vi "Combination_Digitizer_Configure.vi"(0 "Mode":T1(ring), 1 "Horizontal Settings":T2={"number of records"=1, "reference position"=50.0, "min record length"=50000, "min sample rate"=200000.0, "enforce realtime"=FALSE, "maximum input frequency"=0.0} {"maximum input frequency" format="%.2f"; "min sample rate" step=1000000.0 format="%.0p"; "reference position" format="%.1f"; "number of records" step=1}, 2 "Vertical Settings":T4={"vertical coupling"=enum."DC", "probe attenuation"=20.0, "vertical range"=120.0, "vertical offset"=0.0} {"vertical offset" format="%.4f"; "vertical range" format="%.2f"; "probe attenuation" format="%.1f"}, 3 "Trigger settings":T3={"trigger level"=30.0, "trigger type"=enum."Edge", "Trigger Source"=enum."Channel 0", "Trigger Slope"=enum."Positive"} {"trigger level" format="%.2f"}, 5 "Channel Name":string="0", 11 "error in":errorcluster) -> (6 "Waveform Array":waveform(dbl)[](array[waveform]), 8 "Ch1_Plot":dbl[](array[numeric]), 15 "error out":errorcluster)   [LabVIEW 2010]
uses:
  <instrlib>/niScope/Controls/niScope trigger slope.ctl
  <instrlib>/niScope/Controls/niScope trigger source.ctl
  <instrlib>/niScope/Controls/niScope export destinations.ctl
  <instrlib>/niScope/Controls/niScope exportable signals.ctl
  <instrlib>/niScope/Controls/niScope trigger source digital.ctl
  <instrlib>/niScope/Configure/Trigger/niScope Configure Trigger Edge.vi
  <instrlib>/niScope/Configure/Trigger/niScope Configure Trigger Digital.vi
  <instrlib>/niScope/Configure/Trigger/niScope Configure Trigger Immediate.vi
  <instrlib>/niScope/Acquire/niScope Multi Read Cluster.vi
  <instrlib>/niScope/Acquire/Fetch/niScope Multi Fetch Cluster.vi
panel:
  out "Waveform":T5(graph)
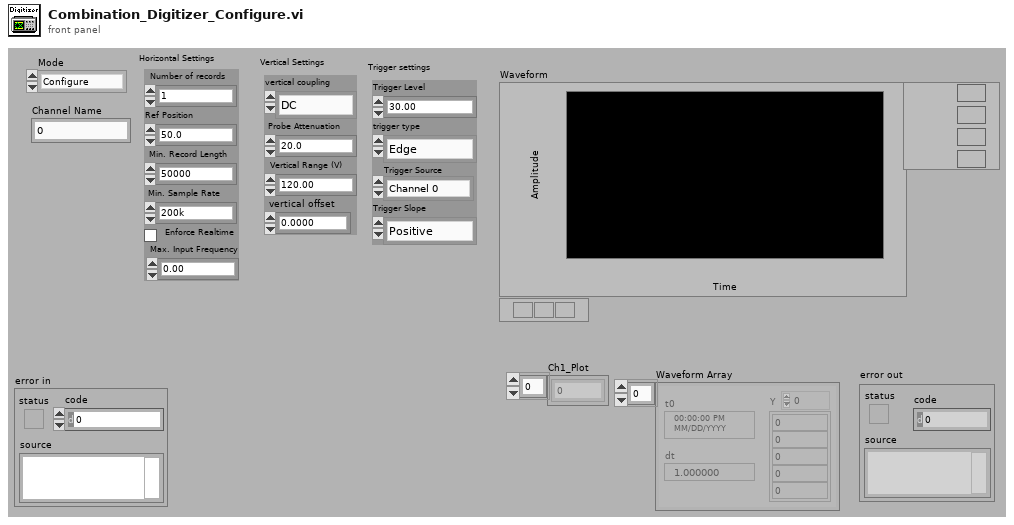
[diagram p1: front panel]
types:
  T1 = enum16{"Configure", "Read", "TriggerRead", "Close", "Init"}
  T2 = cluster{"number of records":i32, "reference position":dbl, "min record length":i32, "min sample rate":dbl, "enforce realtime":bool, "maximum input frequency":dbl}
  T3 = cluster{"trigger level":dbl, "trigger type":enum16{"Edge", "Digital", "Immediate"}, "Trigger Source":enum8{"Immediate", "Channel 0", "Channel 1", "Channel 2", "Channel 3", "Channel 4", "Channel 5", "Channel 6", "Channel 7", "External TRIG", "Software Trigger", "RTSI 0", "RTSI 1", "RTSI 2", "RTSI 3", "RTSI 4", "RTSI 5", "RTSI 6", "PFI 0", "PFI 1", "PFI 2", "PXI Star Trigger"}, "Trigger Slope":enum16{"Positive", "Negative"}}
  T4 = cluster{"vertical coupling":enum16{"AC", "DC", "Ground"}, "probe attenuation":dbl, "vertical range":dbl, "vertical offset":dbl}
  T5 = cluster{"relativeInitialX":dbl, "xIncrement":dbl, "wfm":dbl[]}[]
  T6 = typedef "niScope trigger source.ctl" = string
  T7 = typedef "niScope trigger source digital.ctl" = string
  T8 = typedef "niScope export destinations.ctl" = string
  T9 = cluster{"Dig1 Channels":string, "Channel1 Scale":dbl, "Dig1 Used":bool, "Dig1 Ref":refnum<k15>, "min record length":i32, "Dig2 Channels":string, "Dig2 Used":bool, "Dig2 Ref":refnum<k15>, "trigger type":enum16{"Edge", "Digital", "Immediate"}}
  T10 = enum8{"Immediate", "Channel 0", "Channel 1", "Channel 2", "Channel 3", "Channel 4", "Channel 5", "Channel 6", "Channel 7", "External TRIG", "Software Trigger", "RTSI 0", "RTSI 1", "RTSI 2", "RTSI 3", "RTSI 4", "RTSI 5", "RTSI 6", "PFI 0", "PFI 1", "PFI 2", "PXI Star Trigger"}
  T11 = typedef "niScope trigger slope.ctl" = i32
  T12 = typedef "niScope exportable signals.ctl" = u16
  T13 = cluster{"relativeInitialX":dbl, "xIncrement":dbl, "wfm":dbl[]}
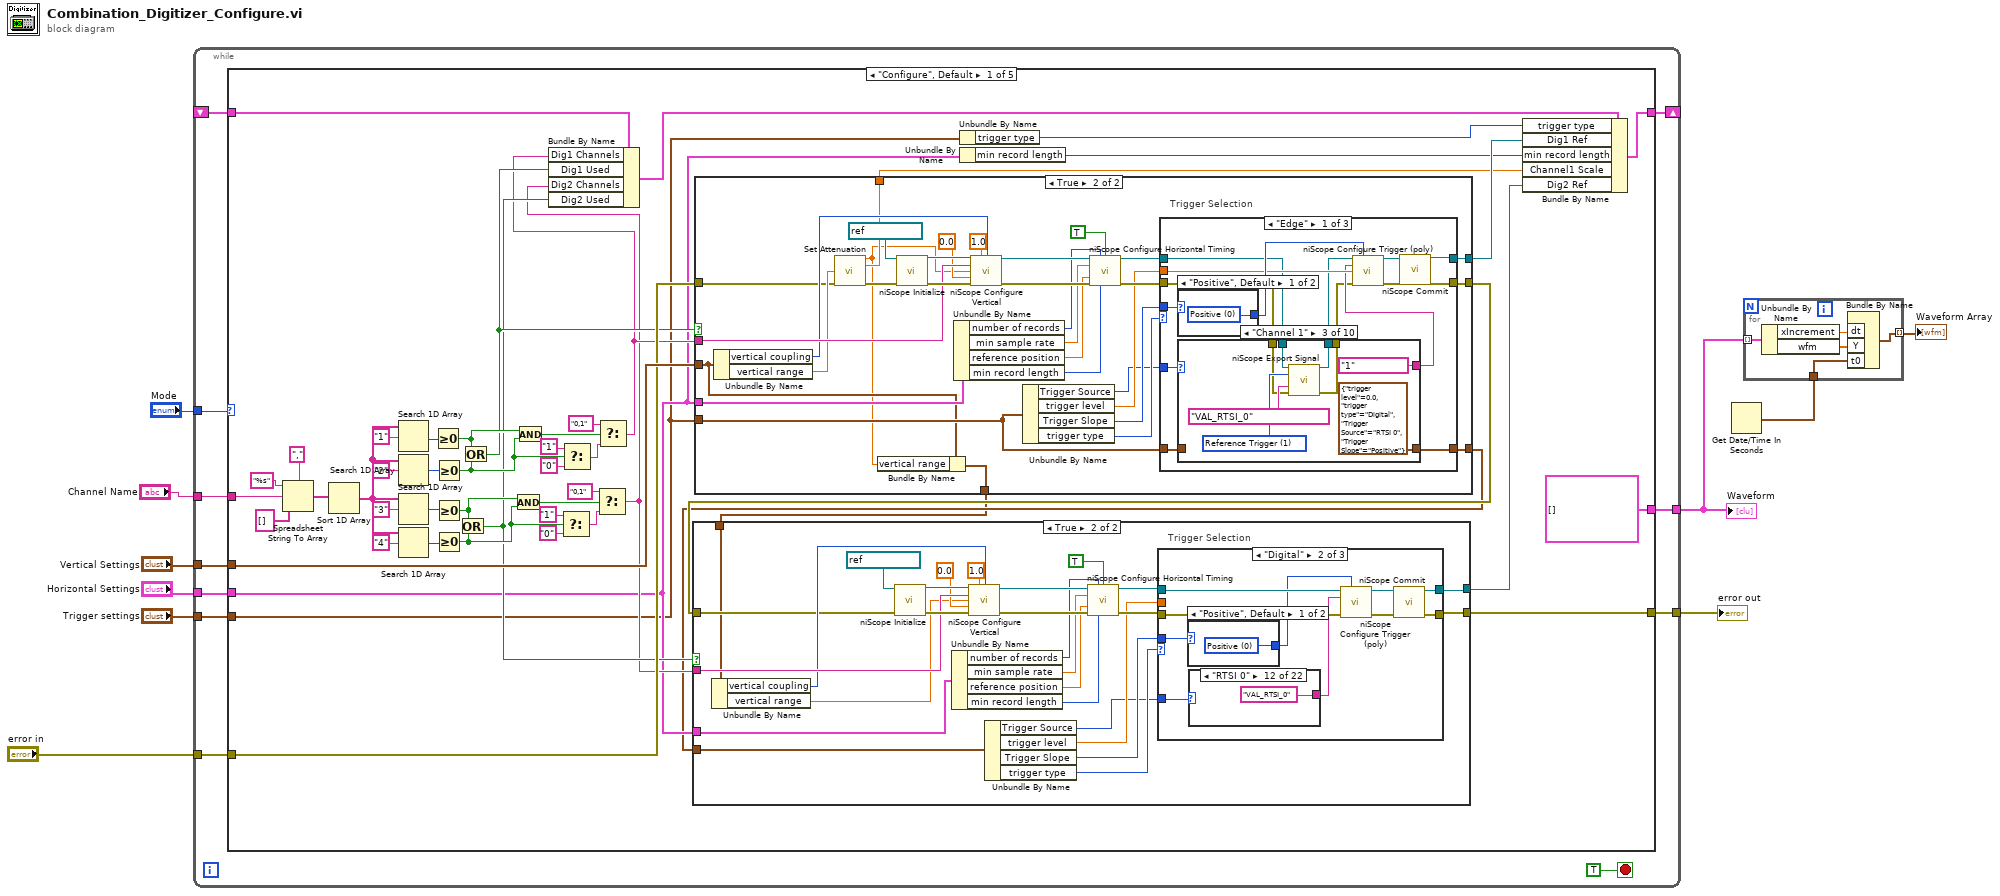
[diagram p0: block diagram]
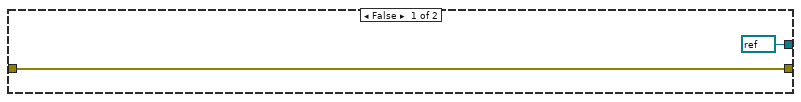
[diagram p2: hidden frame]
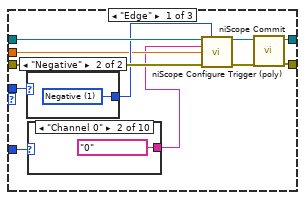
[diagram p3: hidden frame]
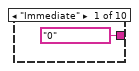
[diagram p4: hidden frame]
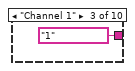
[diagram p5: hidden frame]
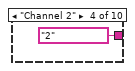
[diagram p6: hidden frame]
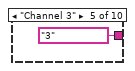
[diagram p7: hidden frame]
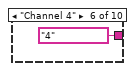
[diagram p8: hidden frame]
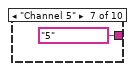
[diagram p9: hidden frame]
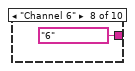
[diagram p10: hidden frame]
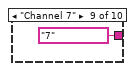
[diagram p11: hidden frame]
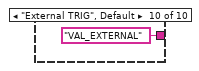
[diagram p12: hidden frame]
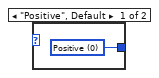
[diagram p13: hidden frame]
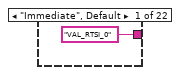
[diagram p14: hidden frame]
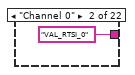
[diagram p15: hidden frame]
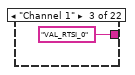
[diagram p16: hidden frame]
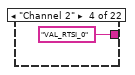
[diagram p17: hidden frame]
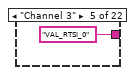
[diagram p18: hidden frame]
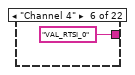
[diagram p19: hidden frame]
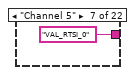
[diagram p20: hidden frame]
diagram:
  n1 = while {
    tunnel: "Mode" -> [w20]
    shift-right: [w14] -> _
    shift-left: _ -> [w19]
    tunnel: "error in" -> [w13]
    tunnel: "Channel Name" -> [w18]
    tunnel: "Vertical Settings" -> [w17]
    tunnel: "Horizontal Settings" -> [w16]
    tunnel: "Trigger settings" -> [w15]
    tunnel: [w12] -> w5
    tunnel: [w11] -> w3
    stop <- TRUE stop-if-true
    n2 = case shown="\"Configure\", Default" w20 {
      tunnel: w19 -> [w38 w307 w410 w437 w486]
      tunnel: w18 -> [w42 _ _ _ _]
      tunnel: w17 -> [w41 _ _ _ _]
      tunnel: w16 -> [w28 _ _ _ _]
      tunnel: w15 -> [w25 _ _ _ _]
      tunnel: [w40 w307 w410 w437 T9 {"Dig1 Channels"="", "Channel1 Scale"=0.0, "Dig1 Used"=FALSE, "Dig1 Ref"="", "min record length"=0, "Dig2 Channels"="", "Dig2 Used"=FALSE, "Dig2 Ref"="", "trigger type"=enum."Immediate"}] -> w14
      tunnel: w13 -> [w39 w313 w413 w443 w489]
      tunnel: [w33 w318 w416 w448 w492] -> w12
      tunnel: [T5 [] w305 T5 [] w436 T5 []] -> w11
      frame "Configure", Default {
        n3 = Spreadsheet String To Array(delimiter (Tab)=",", format string="%s", spreadsheet string=w42, array type (2D Dbl)=string[] []) -> (array=w67:string[])
        n4 = Sort 1D Array(array=w67) -> (sorted array=w66:string[])
        n5 = Search 1D Array(1D array=w66, element="1") -> (index of element=w61:i32)  [unwired: 1 in]
        n6 = Search 1D Array(1D array=w66, element="2") -> (index of element=w58:i32)  [unwired: 1 in]
        n7 = Search 1D Array(1D array=w66, element="3") -> (index of element=w59:i32)  [unwired: 1 in]
        n8 = Search 1D Array(1D array=w66, element="4") -> (index of element=w60:i32)  [unwired: 1 in]
        n9 = Greater Or Equal To 0?(x=w61) -> (x >= 0?=w57:bool)
        n10 = Greater Or Equal To 0?(x=w58) -> (x >= 0?=w53:bool)
        n11 = Greater Or Equal To 0?(x=w59) -> (x >= 0?=w56:bool)
        n12 = Greater Or Equal To 0?(x=w60) -> (x >= 0?=w44:bool)
        n13 = Or(x=w56, y=w44) -> (x .or. y?=w31:bool)
        n14 = Or(x=w57, y=w53) -> (x .or. y?=w32:bool)
        n15 = And(x=w56, y=w44) -> (x .and. y?=w45:bool)
        n16 = And(x=w57, y=w53) -> (x .and. y?=w55:bool)
        n17 = Select(t="1", s=w44, f="0") -> (s? t:f=w47:string)
        n18 = Select(t="1", s=w53, f="0") -> (s? t:f=w51:string)
        n19 = Select(t="0,1", s=w45, f=w47) -> (s? t:f=w29:string)
        n20 = Select(t="0,1", s=w55, f=w51) -> (s? t:f=w30:string)
        n21 = Bundle By Name(cluster=w38, "Dig1 Channels"=w30, "Dig1 Used"=w32, "Dig2 Channels"=w29, "Dig2 Used"=w31) -> (w37:T9)
        n22 = case shown="True" w32 {
          tunnel: [w165 w193] -> w43
          tunnel: w39 -> [w165 w187]
          tunnel: w30 -> [_ w191]
          tunnel: w41 -> [w161 w168]
          tunnel: w28 -> [_ w182]
          tunnel: w25 -> [w162 w170]
          tunnel: [refnum<k15> refnum ("instrument handle out") w176] -> w36
          tunnel: [1.0 ("Gain Multiplier") w174] -> w34
          tunnel: [w162 w169] -> w23
          tunnel: [w161 w166] -> w22
          frame False {
          }
          frame True {
            n23 = Unbundle By Name(w168) -> ("vertical coupling"=w190:enum16{"AC", "DC", "Ground"}, "vertical range"=w188:dbl)
            n24 = call "Set Attenuation.vi"("vertical range"=w188, "error in"=w187) -> ("Requested Range"=w167:dbl, "Gain Multiplier"=w174:dbl, "error out"=w186:errorcluster)  [unwired: 11 in]
            n25 = Bundle By Name(cluster=w168, "vertical range"=w167) -> (w166:T4)
            n26 = call <instrlib>:"niScope Initialize.vi"("resource name"=refnum<k15> "PXI1Slot6", "error in"=w186) -> ("instrument handle"=w197:refnum<k15>, "error out"=w194:errorcluster)  [unwired: 12 in]
            n27 = Unbundle By Name(w182) -> ("number of records"=w181:i32, "min sample rate"=w180:dbl, "reference position"=w179:dbl, "min record length"=w178:i32)
            n28 = call <instrlib>:"niScope Configure Vertical.vi"("instrument handle"=w197, "probe attenuation"=1.0, "vertical coupling"=w190, "channels"=w191, "vertical range"=w167, "vertical offset"=0.0, "error in"=w194) -> ("instrument handle out"=w184:refnum<k15>, "error out"=w183:errorcluster)  [unwired: 7 in]
            n29 = Unbundle By Name(w170) -> ("Trigger Source"=w171:T10, "trigger level"=w177:dbl, "Trigger Slope"=w172:enum16{"Positive", "Negative"}, "trigger type"=w173:enum16{"Edge", "Digital", "Immediate"})
            n30 = call <instrlib>:"niScope Configure Horizontal Timing.vi"("instrument handle"=w184, "number of records"=w181, "enforce realtime"=TRUE, "min sample rate"=w180, "reference position"=w179, "error in"=w183, "min record length"=w178) -> ("instrument handle out"=w195:refnum<k15>, "error out"=w196:errorcluster)  [unwired: 7 in]
            n31 = case "Trigger Selection" shown="\"Edge\"" w173 {
              tunnel: w196 -> [w199 w271 w300]
              tunnel: [w204 w264 w297] -> w193
              tunnel: w195 -> [w201 w270 w299]
              tunnel: [w205 w265 w298] -> w176
              tunnel: w171 -> [w209 w267 _]
              tunnel: w177 -> [w210 _ _]
              tunnel: w172 -> [w212 w269 _]
              tunnel: w170 -> [w203 w263 w296]
              tunnel: [w202 w263 w296] -> w169
              frame "Edge" {
                n32 = case shown="\"Positive\", Default" w212 {
                  tunnel: [w261 w262] -> w211
                  frame "Positive", Default {
                    w261 = T11 0 items=["Positive", "Negative"] ("trigger slope")
                  }
                  frame "Negative" {
                    w262 = T11 1 items=["Positive", "Negative"] ("trigger slope")
                  }
                }
                n33 = case shown="\"Channel 1\"" w209 {
                  tunnel: [T6 "0" ("trigger source") T6 "0" ("trigger source") T6 "1" ("trigger source") T6 "2" ("trigger source") T6 "3" ("trigger source") T6 "4" ("trigger source") T6 "5" ("trigger source") T6 "6" ("trigger source") T6 "7" ("trigger source") T6 "VAL_EXTERNAL" ("trigger source")] -> w208
                  tunnel: w203 -> [w215 _ _ w235 w239 w243 w247 w251 w255 w259]
                  tunnel: [w215 T3 {"trigger level"=0.0, "trigger type"=enum."Digital", "Trigger Source"=enum."RTSI 0", "Trigger Slope"=enum."Positive"} ("Trigger settings") T3 {"trigger level"=0.0, "trigger type"=enum."Digital", "Trigger Source"=enum."RTSI 0", "Trigger Slope"=enum."Positive"} ("Trigger settings") w235 w239 w243 w247 w251 w255 w259] -> w202
                  tunnel: w201 -> [w214 w220 w228 w234 w238 w242 w246 w250 w254 w258]
                  tunnel: [w214 w218 w227 w234 w238 w242 w246 w250 w254 w258] -> w200
                  tunnel: w199 -> [w213 w219 w226 w233 w237 w241 w245 w249 w253 w257]
                  tunnel: [w213 w217 w225 w233 w237 w241 w245 w249 w253 w257] -> w198
                  frame "Immediate" {
                  }
                  frame "Channel 0" {
                    w221 = T12 1 items=["None"=0, "Start Trigger"=2, "Advance Trigger"=5, "Reference Trigger"=1, "End of Record Event"=4, "End of Acquisition Event"=3, "Ready for Start Event"=7, "Ready for Advance Event"=6, "Ready for Reference Event"=10, "Reference Clock"=100, "Sample Clock"=101, "5 Volt Power"=13] ("signal")
                    n34 = call <instrlib>:"niScope Export Signal.vi"("instrument handle"=w220, "signal"=w221, "output terminal"=T8 "VAL_RTSI_0", "error in"=w219) -> ("instrument handle out"=w218:refnum<k15>, "error out"=w217:errorcluster)  [unwired: 10 in]
                  }
                  frame "Channel 1" {
                    w229 = T12 1 items=["None"=0, "Start Trigger"=2, "Advance Trigger"=5, "Reference Trigger"=1, "End of Record Event"=4, "End of Acquisition Event"=3, "Ready for Start Event"=7, "Ready for Advance Event"=6, "Ready for Reference Event"=10, "Reference Clock"=100, "Sample Clock"=101, "5 Volt Power"=13] ("signal")
                    n35 = call <instrlib>:"niScope Export Signal.vi"("instrument handle"=w228, "signal"=w229, "output terminal"=T8 "VAL_RTSI_0", "error in"=w226) -> ("instrument handle out"=w227:refnum<k15>, "error out"=w225:errorcluster)  [unwired: 10 in]
                  }
                  frame "Channel 2" {
                  }
                  frame "Channel 3" {
                  }
                  frame "Channel 4" {
                  }
                  frame "Channel 5" {
                  }
                  frame "Channel 6" {
                  }
                  frame "Channel 7" {
                  }
                  frame "External TRIG", Default {
                  }
                }
                n36 = call-poly <instrlib>:"niScope Configure Trigger (poly).vi"("instrument handle"=w200, "trigger slope"=w211, "trigger source"=w208, "trigger level"=w210, "error in"=w198) -> ("instrument handle out"=w207:refnum<k15>, "error out"=w206:errorcluster)  [unwired: 9 in]
                n37 = call <instrlib>:"niScope Commit.vi"("instrument handle"=w207, "error in"=w206) -> ("instrument handle out"=w205:refnum<k15>, "error out"=w204:errorcluster)  [unwired: 12 in]
              }
              frame "Digital" {
                n38 = case shown="\"Negative\"" w269 {
                  tunnel: [w294 w295] -> w268
                  frame "Positive", Default {
                    w294 = T11 0 items=["Positive", "Negative"] ("trigger slope")
                  }
                  frame "Negative" {
                    w295 = T11 1 items=["Positive", "Negative"] ("trigger slope")
                  }
                }
                n39 = case shown="\"PXI Star Trigger\"" w267 {
                  tunnel: [T7 "VAL_RTSI_0" ("trigger source") T7 "VAL_RTSI_0" ("trigger source") T7 "VAL_RTSI_0" ("trigger source") T7 "VAL_RTSI_0" ("trigger source") T7 "VAL_RTSI_0" ("trigger source") T7 "VAL_RTSI_0" ("trigger source") T7 "VAL_RTSI_0" ("trigger source") T7 "VAL_RTSI_0" ("trigger source") T7 "VAL_RTSI_0" ("trigger source") T7 "VAL_RTSI_0" ("trigger source") T7 "VAL_RTSI_0" ("trigger source") T7 "VAL_RTSI_0" ("trigger source") T7 "VAL_RTSI_1" ("trigger source") T7 "VAL_RTSI_2" ("trigger source") T7 "VAL_RTSI_3" ("trigger source") T7 "VAL_RTSI_4" ("trigger source") T7 "VAL_RTSI_5" ("trigger source") T7 "VAL_RTSI_6" ("trigger source") T7 "VAL_PFI_0" ("trigger source") T7 "VAL_PFI_1" ("trigger source") T7 "VAL_PFI_2" ("trigger source") T7 "VAL_PXI_STAR" ("trigger source")] -> w266
                  frame "Immediate", Default {
                  }
                  frame "Channel 0" {
                  }
                  frame "Channel 1" {
                  }
                  frame "Channel 2" {
                  }
                  frame "Channel 3" {
                  }
                  frame "Channel 4" {
                  }
                  frame "Channel 5" {
                  }
                  frame "Channel 6" {
                  }
                  frame "Channel 7" {
                  }
                  frame "External TRIG" {
                  }
                  frame "Software Trigger" {
                  }
                  frame "RTSI 0" {
                  }
                  frame "RTSI 1" {
                  }
                  frame "RTSI 2" {
                  }
                  frame "RTSI 3" {
                  }
                  frame "RTSI 4" {
                  }
                  frame "RTSI 5" {
                  }
                  frame "RTSI 6" {
                  }
                  frame "PFI 0" {
                  }
                  frame "PFI 1" {
                  }
                  frame "PFI 2" {
                  }
                  frame "PXI Star Trigger" {
                  }
                }
                n40 = call-poly <instrlib>:"niScope Configure Trigger (poly).vi"("instrument handle"=w270, "trigger slope"=w268, "trigger source"=w266, "error in"=w271) -> ("instrument handle out"=w265:refnum<k15>, "error out"=w264:errorcluster)  [unwired: 10 in]
              }
              frame "Immediate", Default {
                n41 = call-poly <instrlib>:"niScope Configure Trigger (poly).vi"("instrument handle"=w299, "error in"=w300) -> ("instrument handle out"=w298:refnum<k15>, "error out"=w297:errorcluster)  [unwired: 12 in]
              }
            }
          }
        }
        n42 = case shown="True" w31 {
          tunnel: [w72 w79] -> w33
          tunnel: w43 -> [w72 w84]
          tunnel: w29 -> [_ w96]
          tunnel: w28 -> [_ w90]
          tunnel: w23 -> [_ w85]
          tunnel: [refnum<k15> refnum ("instrument handle out") w80] -> w35
          tunnel: w22 -> [_ w73]
          frame False {
          }
          frame True {
            n43 = Unbundle By Name(w73) -> ("vertical coupling"=w95:enum16{"AC", "DC", "Ground"}, "vertical range"=w83:dbl)
            n44 = call <instrlib>:"niScope Initialize.vi"("resource name"=refnum<k15> "PXI1Slot4", "error in"=w84) -> ("instrument handle"=w99:refnum<k15>, "error out"=w98:errorcluster)  [unwired: 12 in]
            n45 = Unbundle By Name(w90) -> ("number of records"=w89:i32, "min sample rate"=w88:dbl, "reference position"=w87:dbl, "min record length"=w86:i32)
            n46 = call <instrlib>:"niScope Configure Vertical.vi"("instrument handle"=w99, "probe attenuation"=1.0, "vertical coupling"=w95, "channels"=w96, "vertical range"=w83, "vertical offset"=0.0, "error in"=w98) -> ("instrument handle out"=w92:refnum<k15>, "error out"=w91:errorcluster)  [unwired: 7 in]
            n47 = Unbundle By Name(w85) -> ("Trigger Source"=w74:T10, "trigger level"=w77:dbl, "Trigger Slope"=w75:enum16{"Positive", "Negative"}, "trigger type"=w76:enum16{"Edge", "Digital", "Immediate"})
            n48 = call <instrlib>:"niScope Configure Horizontal Timing.vi"("instrument handle"=w92, "number of records"=w89, "enforce realtime"=TRUE, "min sample rate"=w88, "reference position"=w87, "error in"=w91, "min record length"=w86) -> ("instrument handle out"=w81:refnum<k15>, "error out"=w78:errorcluster)  [unwired: 7 in]
            n49 = case "Trigger Selection" shown="\"Digital\"" w76 {
              tunnel: w78 -> [w110 w132 w160]
              tunnel: [w100 w123 w157] -> w79
              tunnel: w81 -> [w109 w131 w159]
              tunnel: [w102 w124 w158] -> w80
              tunnel: w74 -> [w105 w128 _]
              tunnel: w77 -> [w106 _ _]
              tunnel: w75 -> [w108 w130 _]
              frame "Edge" {
                n50 = case shown="\"Negative\"" w108 {
                  tunnel: [w121 w122] -> w107
                  frame "Positive", Default {
                    w121 = T11 0 items=["Positive", "Negative"] ("trigger slope")
                  }
                  frame "Negative" {
                    w122 = T11 1 items=["Positive", "Negative"] ("trigger slope")
                  }
                }
                n51 = case shown="\"Channel 0\"" w105 {
                  tunnel: [T6 "0" ("trigger source") T6 "0" ("trigger source") T6 "1" ("trigger source") T6 "2" ("trigger source") T6 "3" ("trigger source") T6 "4" ("trigger source") T6 "5" ("trigger source") T6 "6" ("trigger source") T6 "7" ("trigger source") T6 "VAL_EXTERNAL" ("trigger source")] -> w104
                  frame "Immediate" {
                  }
                  frame "Channel 0" {
                  }
                  frame "Channel 1" {
                  }
                  frame "Channel 2" {
                  }
                  frame "Channel 3" {
                  }
                  frame "Channel 4" {
                  }
                  frame "Channel 5" {
                  }
                  frame "Channel 6" {
                  }
                  frame "Channel 7" {
                  }
                  frame "External TRIG", Default {
                  }
                }
                n52 = call-poly <instrlib>:"niScope Configure Trigger (poly).vi"("instrument handle"=w109, "trigger slope"=w107, "trigger source"=w104, "trigger level"=w106, "error in"=w110) -> ("instrument handle out"=w103:refnum<k15>, "error out"=w101:errorcluster)  [unwired: 9 in]
                n53 = call <instrlib>:"niScope Commit.vi"("instrument handle"=w103, "error in"=w101) -> ("instrument handle out"=w102:refnum<k15>, "error out"=w100:errorcluster)  [unwired: 12 in]
              }
              frame "Digital" {
                n54 = case shown="\"Positive\", Default" w130 {
                  tunnel: [w155 w156] -> w129
                  frame "Positive", Default {
                    w155 = T11 0 items=["Positive", "Negative"] ("trigger slope")
                  }
                  frame "Negative" {
                    w156 = T11 1 items=["Positive", "Negative"] ("trigger slope")
                  }
                }
                n55 = case shown="\"RTSI 0\"" w128 {
                  tunnel: [T7 "VAL_RTSI_0" ("trigger source") T7 "VAL_RTSI_0" ("trigger source") T7 "VAL_RTSI_0" ("trigger source") T7 "VAL_RTSI_0" ("trigger source") T7 "VAL_RTSI_0" ("trigger source") T7 "VAL_RTSI_0" ("trigger source") T7 "VAL_RTSI_0" ("trigger source") T7 "VAL_RTSI_0" ("trigger source") T7 "VAL_RTSI_0" ("trigger source") T7 "VAL_RTSI_0" ("trigger source") T7 "VAL_RTSI_0" ("trigger source") T7 "VAL_RTSI_0" ("trigger source") T7 "VAL_RTSI_1" ("trigger source") T7 "VAL_RTSI_2" ("trigger source") T7 "VAL_RTSI_3" ("trigger source") T7 "VAL_RTSI_4" ("trigger source") T7 "VAL_RTSI_5" ("trigger source") T7 "VAL_RTSI_6" ("trigger source") T7 "VAL_PFI_0" ("trigger source") T7 "VAL_PFI_1" ("trigger source") T7 "VAL_PFI_2" ("trigger source") T7 "VAL_PXI_STAR" ("trigger source")] -> w127
                  frame "Immediate", Default {
                  }
                  frame "Channel 0" {
                  }
                  frame "Channel 1" {
                  }
                  frame "Channel 2" {
                  }
                  frame "Channel 3" {
                  }
                  frame "Channel 4" {
                  }
                  frame "Channel 5" {
                  }
                  frame "Channel 6" {
                  }
                  frame "Channel 7" {
                  }
                  frame "External TRIG" {
                  }
                  frame "Software Trigger" {
                  }
                  frame "RTSI 0" {
                  }
                  frame "RTSI 1" {
                  }
                  frame "RTSI 2" {
                  }
                  frame "RTSI 3" {
                  }
                  frame "RTSI 4" {
                  }
                  frame "RTSI 5" {
                  }
                  frame "RTSI 6" {
                  }
                  frame "PFI 0" {
                  }
                  frame "PFI 1" {
                  }
                  frame "PFI 2" {
                  }
                  frame "PXI Star Trigger" {
                  }
                }
                n56 = call-poly <instrlib>:"niScope Configure Trigger (poly).vi"("instrument handle"=w131, "trigger slope"=w129, "trigger source"=w127, "error in"=w132) -> ("instrument handle out"=w126:refnum<k15>, "error out"=w125:errorcluster)  [unwired: 10 in]
                n57 = call <instrlib>:"niScope Commit.vi"("instrument handle"=w126, "error in"=w125) -> ("instrument handle out"=w124:refnum<k15>, "error out"=w123:errorcluster)  [unwired: 12 in]
              }
              frame "Immediate", Default {
                n58 = call-poly <instrlib>:"niScope Configure Trigger (poly).vi"("instrument handle"=w159, "error in"=w160) -> ("instrument handle out"=w158:refnum<k15>, "error out"=w157:errorcluster)  [unwired: 12 in]
              }
            }
          }
        }
        n59 = Unbundle By Name(w25) -> ("trigger type"=w24:enum16{"Edge", "Digital", "Immediate"})
        n60 = Unbundle By Name(w28) -> ("min record length"=w27:i32)
        n61 = Bundle By Name(cluster=w37, "trigger type"=w24, "Dig1 Ref"=w36, "min record length"=w27, "Channel1 Scale"=w34, "Dig2 Ref"=w35) -> (w40:T9)
      }
      frame "Read" {
        n62 = Unbundle By Name(w307) -> ("trigger type"=w302:enum16{"Edge", "Digital", "Immediate"}, "Dig1 Used"=w317:bool, "Dig1 Ref"=w316:refnum<k15>, "Dig1 Channels"=w315:string, "min record length"=w314:i32, "Channel1 Scale"=w308:dbl)
        n63 = Unbundle By Name(w307) -> ("trigger type"=w301:enum16{"Edge", "Digital", "Immediate"}, "Dig2 Used"=w312:bool, "Dig2 Ref"=w311:refnum<k15>, "Dig2 Channels"=w310:string, "min record length"=w309:i32)
        n64 = case shown="True" w317 {
          tunnel: w315 -> [_ w381]
          tunnel: w313 -> [w375 w379]
          tunnel: w316 -> [_ w382]
          tunnel: [w375 w377] -> w319
          tunnel: [T5 [] ("waveform") w378] -> w320
          tunnel: w314 -> [_ w380]
          tunnel: w302 -> [_ w376]
          frame False {
          }
          frame True {
            n65 = case shown="\"Digital\", Default" w376 {
              tunnel: w382 -> [w389 w399]
              tunnel: w381 -> [w388 w398]
              tunnel: w380 -> [w387 w397]
              tunnel: w379 -> [w386 w396]
              tunnel: [w384 w391] -> w378
              tunnel: [w383 w394] -> w377
              frame "Immediate" {
                n66 = call-poly <instrlib>:"niScope Read (poly).vi"("timeout"=10.0, "error in"=w386, "numSamples"=w387, "channels"=w388, "instrument handle"=w389) -> ("error out"=w383:errorcluster, "waveform"=w384:T5)  [unwired: 3 in, 2 out]
              }
              frame "Digital", Default {
                n67 = call-poly <instrlib>:"niScope Fetch (poly).vi"("timeout"=10.0, "error in"=w396, "numSamples"=w397, "channels"=w398, "instrument handle"=w399) -> ("error out"=w393:errorcluster, "waveform"=w392:T5, "instrument handle out"=w390:refnum<k15>)  [unwired: 3 in, 1 out]
                n68 = case shown="Error" w393 {
                  tunnel: w393 -> [w400 w406]
                  tunnel: [w400 w403] -> w394
                  tunnel: w392 -> [w401 _]
                  tunnel: [w401 T5 [{"relativeInitialX"=0.0, "xIncrement"=0.0, "wfm"=[]}, {"relativeInitialX"=0.0, "xIncrement"=0.0, "wfm"=[]}] ("waveform")] -> w391
                  tunnel: w390 -> [_ w402]
                  frame No Error {
                  }
                  frame Error {
                    n69 = call <vilib>:"Clear Errors.vi"("error in (no error)"=w406) -> ("error out"=w404:errorcluster)  [unwired: 6 in]
                    n70 = call <instrlib>:"niScope Abort.vi"("instrument handle"=w402, "error in"=w404) -> ("error out"=w403:errorcluster)  [unwired: 12 in, 1 out]
                  }
                }
              }
            }
          }
        }
        n71 = case shown="True" w312 {
          tunnel: w310 -> [_ w346]
          tunnel: w319 -> [w342 w344]
          tunnel: w311 -> [_ w347]
          tunnel: w309 -> [_ w345]
          tunnel: [w342 w349] -> w318
          tunnel: [T5 [] ("waveform") w348] -> w323
          tunnel: w301 -> [_ w343]
          frame False {
          }
          frame True {
            n72 = case shown="\"Digital\", Default" w343 {
              tunnel: w347 -> [w356 w366]
              tunnel: w346 -> [w355 w365]
              tunnel: w345 -> [w354 w364]
              tunnel: w344 -> [w353 w363]
              tunnel: [w351 w359] -> w348
              tunnel: [w350 w360] -> w349
              frame "Immediate" {
                n73 = call-poly <instrlib>:"niScope Read (poly).vi"("timeout"=10.0, "error in"=w353, "numSamples"=w354, "channels"=w355, "instrument handle"=w356) -> ("error out"=w350:errorcluster, "waveform"=w351:T5)  [unwired: 3 in, 2 out]
              }
              frame "Digital", Default {
                n74 = call-poly <instrlib>:"niScope Fetch (poly).vi"("timeout"=10.0, "error in"=w363, "numSamples"=w364, "channels"=w365, "instrument handle"=w366) -> ("error out"=w358:errorcluster, "waveform"=w361:T5, "instrument handle out"=w357:refnum<k15>)  [unwired: 3 in, 1 out]
                n75 = case shown="Error" w358 {
                  tunnel: w358 -> [w367 w373]
                  tunnel: [w367 w369] -> w360
                  tunnel: w361 -> [w368 _]
                  tunnel: [w368 T5 [{"relativeInitialX"=0.0, "xIncrement"=0.0, "wfm"=[]}, {"relativeInitialX"=0.0, "xIncrement"=0.0, "wfm"=[]}] ("waveform")] -> w359
                  tunnel: w357 -> [_ w371]
                  frame No Error {
                  }
                  frame Error {
                    n76 = call <vilib>:"Clear Errors.vi"("error in (no error)"=w373) -> ("error out"=w370:errorcluster)  [unwired: 6 in]
                    n77 = call <instrlib>:"niScope Abort.vi"("instrument handle"=w371, "error in"=w370) -> ("error out"=w369:errorcluster)  [unwired: 12 in, 1 out]
                  }
                }
              }
            }
          }
        }
        n78 = Greater?(x=w308, y=1.0) -> (0:w322:bool)
        n79 = case shown="True" w322 {
          tunnel: w320 -> [w326 w340]
          tunnel: w308 -> [_ w327]
          tunnel: w323 -> [w325 w333]
          tunnel: [w324 w332] -> w305
          frame False {
            n80 = Build Array (concatenate)(w326, w325) -> (w324:T5)
          }
          frame True {
            # "Add scaling from TEGAM, if used"
            n81 = Index Array(array=w340, index #1=0 ("index"), index #2=1 ("index")) -> (element #1=w337:T13, element #2=w329:T13)
            n82 = Unbundle By Name(w337) -> ("wfm"=w339:dbl[])
            n83 = Unbundle By Name(w329) -> ("wfm"=w331:dbl[])
            n84 = Multiply(x=w339, y=w327) -> (x*y=w336:dbl[])
            n85 = Multiply(x=w331, y=w327) -> (x*y=w330:dbl[])
            n86 = Bundle By Name(cluster=w337, "wfm"=w336) -> (w334:T13)
            n87 = Bundle By Name(cluster=w329, "wfm"=w330) -> (w328:T13)
            n88 = Build Array (concatenate)(w334, w328, w333) -> (w332:T5)
          }
        }
        n89 = Index Array(array=w305, index=0) -> (element=w304:T13)
        n90 = Unbundle By Name(w304) -> ("wfm"=→"Ch1_Plot":dbl[])
      }
      frame "Init" {
        n91 = Unbundle By Name(w410) -> ("trigger type"=w409:enum16{"Edge", "Digital", "Immediate"}, "Dig1 Used"=w415:bool, "Dig1 Ref"=w414:refnum<k15>)
        n92 = Unbundle By Name(w410) -> ("trigger type"=w408:enum16{"Edge", "Digital", "Immediate"}, "Dig2 Used"=w412:bool, "Dig2 Ref"=w411:refnum<k15>)
        n93 = case shown="True" w415 {
          tunnel: w413 -> [w427 w430]
          tunnel: w414 -> [_ w431]
          tunnel: [w427 w429] -> w417
          tunnel: w409 -> [_ w428]
          frame False {
          }
          frame True {
            n94 = case shown="\"Digital\", Default" w428 {
              tunnel: w431 -> [_ w434]
              tunnel: w430 -> [w432 w433]
              tunnel: [w432 w435] -> w429
              frame "Immediate" {
              }
              frame "Digital", Default {
                n95 = call <instrlib>:"niScope Initiate Acquisition.vi"("instrument handle"=w434, "error in"=w433) -> ("error out"=w435:errorcluster)  [unwired: 12 in, 1 out]
              }
            }
          }
        }
        n96 = case shown="True" w412 {
          tunnel: w417 -> [w418 w420]
          tunnel: w411 -> [_ w421]
          tunnel: [w418 w422] -> w416
          tunnel: w408 -> [_ w419]
          frame False {
          }
          frame True {
            n97 = case shown="\"Digital\", Default" w419 {
              tunnel: w421 -> [_ w425]
              tunnel: w420 -> [w423 w424]
              tunnel: [w423 w426] -> w422
              frame "Immediate" {
              }
              frame "Digital", Default {
                n98 = call <instrlib>:"niScope Initiate Acquisition.vi"("instrument handle"=w425, "error in"=w424) -> ("error out"=w426:errorcluster)  [unwired: 12 in, 1 out]
              }
            }
          }
        }
      }
      frame "TriggerRead" {
        n99 = Unbundle By Name(w437) -> ("Dig1 Used"=w447:bool, "Dig1 Ref"=w446:refnum<k15>, "Dig1 Channels"=w445:string, "min record length"=w444:i32, "Channel1 Scale"=w438:dbl)
        n100 = Unbundle By Name(w437) -> ("Dig2 Used"=w442:bool, "Dig2 Ref"=w441:refnum<k15>, "Dig2 Channels"=w440:string, "min record length"=w439:i32)
        n101 = case shown="True" w447 {
          tunnel: w445 -> [_ w482]
          tunnel: w443 -> [w477 w483]
          tunnel: w446 -> [_ w481]
          tunnel: [w477 w478] -> w449
          tunnel: [T5 [] ("waveform") w480] -> w450
          tunnel: w444 -> [_ w479]
          frame False {
          }
          frame True {
            n102 = call-poly <instrlib>:"niScope Read (poly).vi"("error in"=w483, "numSamples"=w479, "channels"=w482, "instrument handle"=w481) -> ("error out"=w478:errorcluster, "waveform"=w480:T5)  [unwired: 4 in, 2 out]
          }
        }
        n103 = case shown="True" w442 {
          tunnel: w440 -> [_ w474]
          tunnel: w449 -> [w469 w475]
          tunnel: w441 -> [_ w473]
          tunnel: w439 -> [_ w472]
          tunnel: [w469 w470] -> w448
          tunnel: [T5 [] ("waveform") w471] -> w453
          frame False {
          }
          frame True {
            n104 = call-poly <instrlib>:"niScope Read (poly).vi"("error in"=w475, "numSamples"=w472, "channels"=w474, "instrument handle"=w473) -> ("error out"=w470:errorcluster, "waveform"=w471:T5)  [unwired: 4 in, 2 out]
          }
        }
        n105 = Greater?(x=w438, y=10.0) -> (0:w452:bool)
        n106 = case shown="True" w452 {
          tunnel: w450 -> [w456 w467]
          tunnel: w438 -> [_ w459]
          tunnel: w453 -> [w455 w458]
          tunnel: [w454 w457] -> w436
          frame False {
            n107 = Build Array (concatenate)(w456, w455) -> (w454:T5)
          }
          frame True {
            # "Add scaling from TEGAM, if used"
            n108 = Index Array(array=w467, index #1=0 ("index"), index #2=1 ("index")) -> (element #1=w464:T13, element #2=w461:T13)
            n109 = Unbundle By Name(w464) -> ("wfm"=w466:dbl[])
            n110 = Multiply(x=w466, y=w459) -> (x*y=w463:dbl[])
            n111 = Bundle By Name(cluster=w464, "wfm"=w463) -> (w460:T13)
            n112 = Build Array (concatenate)(w460, w461, w458) -> (w457:T5)
          }
        }
      }
      frame "Close" {
        n113 = Unbundle By Name(w486) -> ("Dig1 Used"=w491:bool, "Dig1 Ref"=w490:refnum<k15>)
        n114 = Unbundle By Name(w486) -> ("Dig2 Used"=w488:bool, "Dig2 Ref"=w487:refnum<k15>)
        n115 = case shown="True" w491 {
          tunnel: w489 -> [w498 w499]
          tunnel: w490 -> [_ w500]
          tunnel: [w498 w501] -> w493
          frame False {
          }
          frame True {
            n116 = call <instrlib>:"niScope Close.vi"("instrument handle"=w500, "error in"=w499) -> ("error out"=w501:errorcluster)  [unwired: 13 in]
          }
        }
        n117 = case shown="True" w488 {
          tunnel: w493 -> [w494 w496]
          tunnel: w487 -> [_ w495]
          tunnel: [w494 w497] -> w492
          frame False {
          }
          frame True {
            n118 = call <instrlib>:"niScope Close.vi"("instrument handle"=w495, "error in"=w496) -> ("error out"=w497:errorcluster)  [unwired: 13 in]
          }
        }
      }
    }
  }
  "error out" <- w5
  "Waveform" <- w3
  n119 = Get Date/Time In Seconds() -> (seconds since 1Jan1904=w1:timestamp)
  n120 = for {
    tunnel: w3 -> [w506] mode=indexing
    tunnel: [w503] -> w2 mode=indexing
    tunnel: w1 -> [w502]
    n121 = Unbundle By Name(w506) -> ("xIncrement"=w505:dbl, "wfm"=w504:dbl[])
    n122 = Bundle By Name("dt"=w505, "Y"=w504, "t0"=w502) -> (w503:waveform(dbl))  [unwired: 1 in]
  }
  "Waveform Array" <- w2
